vi "Read Active VI.vi"(8 "error in (no error)":errorcluster, 11 "Panel Actor in":refnum<class "Panel Actor.lvclass">) -> (0 "error out":errorcluster, 2 "Active VI ref":refnum<vi>, 3 "Panel Actor out":refnum<class "Panel Actor.lvclass">)   [LabVIEW 2023, in "Panel Actor.lvlib" / "Panel Actor.lvclass"]
doc: "Gets the actor VI ref. If no actove VI has been set, this opens a references to the most specific version of Actor Core.\n----\nPlease see the following web address for additional documentation and tutorial information:\nhttp://www.mooregoodideas.com/mgi-panel-manager/\n\nAuthor: Derek Trepanier\n\nCopyright (c) 2018, Moore Good Ideas, Inc.\n\nAll rights reserved.\n\nRedistribution and use in source and binary forms, with or without modification, are permitted provided that the following conditions are met:\n\n * Redistributions of source code must retain the above copyright notice, this list of conditions and the following disclaimer.\n * Redistributions in binary form must reproduce the above copyright notice, this list of conditions and the following disclaimer in the documentation and/or other materials provided with the distribution.\n * Neither the name of Moore Good Ideas, Inc. nor the names of its contributors may be used to endorse or promote products derived from this software without specific prior written permission.\n\nTHIS SOFTWARE IS PROVIDED BY THE COPYRIGHT HOLDERS AND CONTRIBUTORS \"AS IS\" AND ANY EXPRESS OR IMPLIED WARRANTIES, INCLUDING, BUT NOT LIMITED TO, THE IMPLIED WARRANTIES OF MERCHANTABILITY AND FITNESS FOR A PARTICULAR PURPOSE ARE DISCLAIMED. IN NO EVENT SHALL THE COPYRIGHT OWNER OR CONTRIBUTORS BE LIABLE FOR ANY DIRECT, INDIRECT, INCIDENTAL, SPECIAL, EXEMPLARY, OR CONSEQUENTIAL DAMAGES (INCLUDING, BUT NOT LIMITED TO, PROCUREMENT OF SUBSTITUTE GOODS OR SERVICES; LOSS OF USE, DATA, OR PROFITS; OR BUSINESS INTERRUPTION) HOWEVER CAUSED AND ON ANY THEORY OF LIABILITY, WHETHER IN CONTRACT, STRICT LIABILITY, OR TORT (INCLUDING NEGLIGENCE OR OTHERWISE) ARISING IN ANY WAY OUT OF THE USE OF THIS SOFTWARE, EVEN IF ADVISED OF THE POSSIBILITY OF SUCH DAMAGE."
uses:
  Library/Panel Actor.lvclass
  Library/Panel Actor.lvclass/Panel Actor.ctl
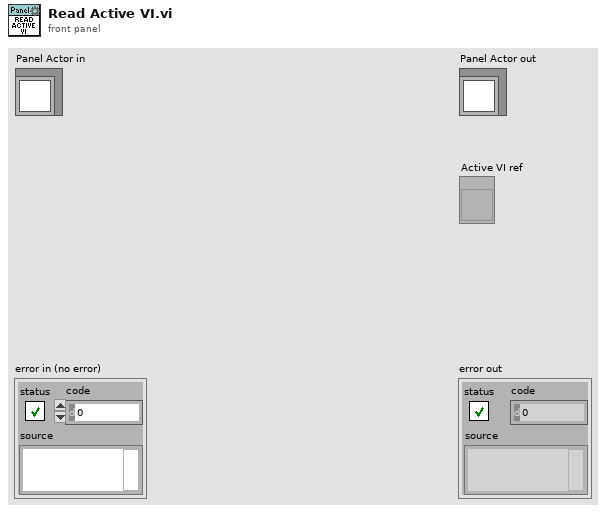
[diagram p1: front panel]
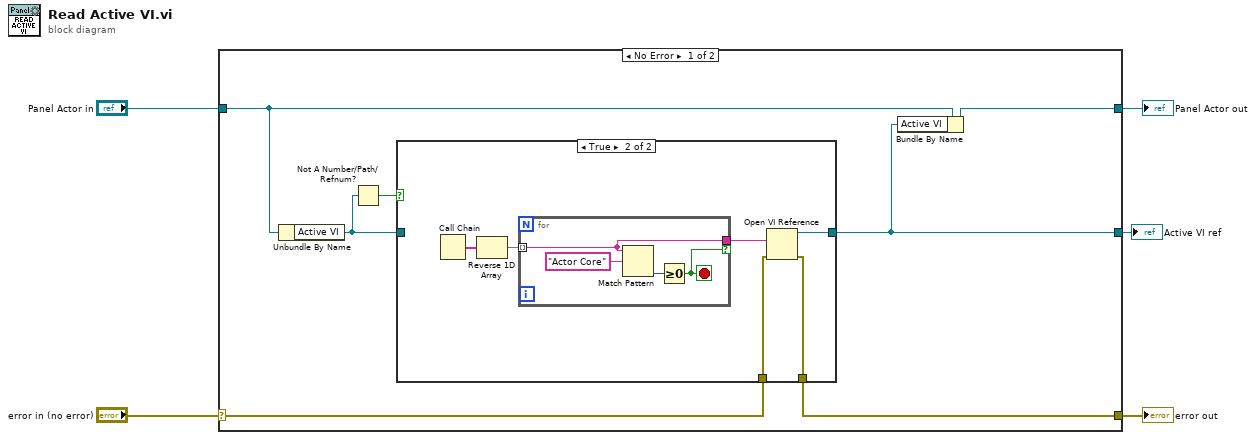
[diagram p0: block diagram]
diagram:
  n1 = case shown="No Error" "error in (no error)" {
    selector: "error in (no error)" -> [w7 w26]
    tunnel: [w6 w26] -> w4
    tunnel: [w9 w25] -> w2
    tunnel: "Panel Actor in" -> [w12 w25]
    tunnel: [w8 _] -> w1
    frame No Error {
      n2 = Unbundle By Name(w12) -> ("Active VI"=w10:refnum<vi>)
      n3 = Not A Number/Path/Refnum?(number/path/refnum=w10) -> (NaN/Path/Refnum?=w11:bool)
      n4 = case shown="True" w11 {
        tunnel: w10 -> [w14 _]
        tunnel: [w14 w17] -> w8
        tunnel: w7 -> [w13 w16]
        tunnel: [w13 w15] -> w6
        frame False {
        }
        frame True {
          n5 = Call Chain() -> (call chain=w20:string[])
          n6 = Reverse 1D Array(array=w20) -> (reversed array=w19:string[])
          n7 = for {
            tunnel: w19 -> [w22] mode=indexing
            tunnel: [w22] -> w18 if=w21
            stop <- w21 stop-if-true
            n8 = Match Pattern(string=w22, regular expression="Actor Core") -> (offset past match=w23:i32)  [unwired: 1 in, 3 out]
            n9 = Greater Or Equal To 0?(x=w23) -> (x >= 0?=w21:bool)
          }
          n10 = Open VI Reference(vi path=w18, error in (no error)=w16) -> (vi reference=w17:refnum<vi>, error out=w15:errorcluster)  [unwired: 4 in]
        }
      }
      n11 = Bundle By Name(cluster=w12, "Active VI"=w8) -> (w9:refnum<class "Panel Actor.lvclass">)
    }
    frame Error {
    }
  }
  "error out" <- w4
  "Panel Actor out" <- w2
  "Active VI ref" <- w1
